vi "Process Current Operation.vi"(8 "error in":errorcluster, 11 "Current Operation in":T1(ring)) -> (0 "error out":errorcluster, 3 "Current Operation out":T1(ring))   [LabVIEW 2023, in "VS Inline Async API.lvlib" / "VS Inline Async API.lvclass"]
uses:
  VS Inline Async API.lvclass
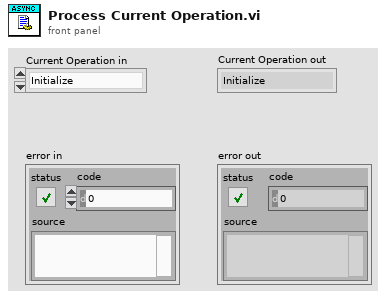
[diagram p1: front panel]
types:
  T1 = enum16{"Initialize", "Start", "Read Data from hardware", "Write Data to hardware", "Close", "Get State"}
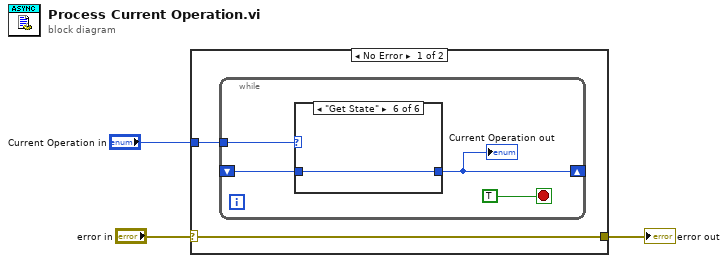
[diagram p0: block diagram]
diagram:
  n1 = case shown="No Error" "error in" {
    selector: "error in" -> [w5 w16]
    tunnel: [w5 w16] -> w2
    tunnel: "Current Operation in" -> [w4 _]
    frame No Error {
      n2 = while {
        tunnel: w4 -> [w8]
        shift-right: [w7] -> _
        shift-left: _ -> [w6]
        stop <- TRUE stop-if-true
        n3 = case shown="\"Get State\"" w8 {
          selector: w8 -> [w10 w11 w12 w13 w14 _]
          tunnel: [w10 w11 w12 w13 w14 w15] -> w7
          tunnel: w6 -> [_ _ _ _ _ w15]
          frame "Initialize", Default {
          }
          frame "Start" {
          }
          frame "Read Data from hardware" {
          }
          frame "Write Data to hardware" {
          }
          frame "Close" {
          }
          frame "Get State" {
          }
        }
        "Current Operation out" <- w7
      }
    }
    frame Error {
    }
  }
  "error out" <- w2
